vi "Send Data.vi"(8 "error in (no error)":errorcluster, 10 "Value":dbl, 11 "Destination":refnum<class "Message Enqueuer.lvclass">) -> (0 "error out":errorcluster)   [LabVIEW 2020, in "Wrapped Actor.lvlib" / "Data Message.lvclass"]
uses:
  Data Message.lvclass
  Data Message.lvclass/Data Message.ctl
  <vilib>/ActorFramework/Self-Addressed Msg/Self-Addressed Msg.lvclass
  C:/Program Files/National Instruments/LabVIEW 2020/vi.lib/ActorFramework/Message/Message.lvclass
  E:/Labview/LV 2020/Libs/Actor Pub Sub/Source/Actor Pub Sub Channels/Pub Sub Event Channel/Data Message/Data Message.lvclass
  <vilib>/ActorFramework/Message Enqueuer/Message Enqueuer.lvclass
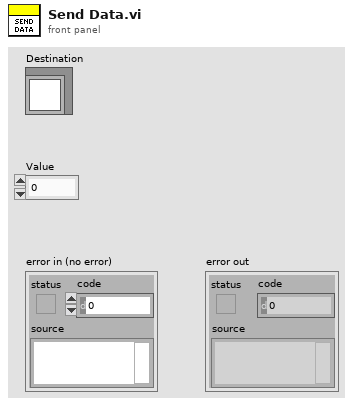
[diagram p1: front panel]
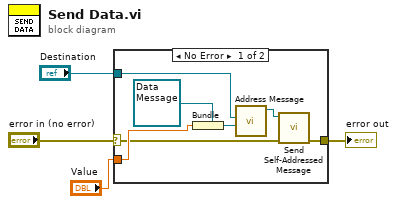
[diagram p0: block diagram]
diagram:
  n1 = case shown="No Error" "error in (no error)" {
    selector: "error in (no error)" -> [w6 w12]
    tunnel: [w5 w12] -> w3
    tunnel: "Destination" -> [w9 _]
    tunnel: "Value" -> [w7 _]
    frame No Error {
      n2 = Bundle(cluster=refnum<class "Data Message.lvclass"> refnum ("Wrapped Actor.lvlib:Data Message.lvclass"), w7) -> (w8:refnum<class "Data Message.lvclass">)
      n3 = call <vilib>:"Address Message.vi"("Message"=w8, "Destination"=w9) -> ("Self-Addressed Message"=w10:refnum<class "Self-Addressed Msg.lvclass">)  [unwired: 9 in]
      n4 = call-dynamic "Send Self-Addressed Message.vi"("error in (no error)"=w6, "Self-Addressed Message in"=w10) -> ("error out"=w5:errorcluster)  [unwired: 8 in, 1 out]
    }
    frame Error {
    }
  }
  "error out" <- w3
